vi "GUI Unit Test.vi"   [LabVIEW 2015]
uses:
  Button_UI/Button_UI.lvclass
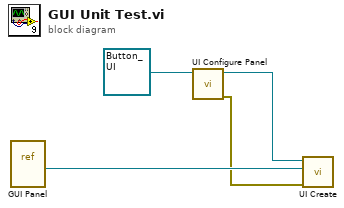
[diagram p0: block diagram]
diagram:
  n1 = vi-ref "GUI Panel.vi"() -> (w4:refnum<vi>)
  n2 = call-dynamic "UI Configure Panel.vi"("Button_UI in"=refnum<class "Button_UI.lvclass"> refnum ("Button_UI")) -> ("error out"=w1:errorcluster, "Button_UI out"=w2:refnum<class "Button_UI.lvclass">)  [unwired: 9 in]
  n3 = call-dynamic "UI Create.vi"("error in (no error)"=w1, "VI Refnum"=w4, "Button_UI in"=w2) -> ()  [unwired: 7 in, 2 out]
